vi "GUI Set Error and Display Error Status.vi"(1 "error in":errorcluster, 2 "Write status only if error occures? (False)":bool, 3 "error name (error)":string="error", 4 "status string name (stat1)":string="stat1") -> ()   [LabVIEW 2013]
doc: "GUI helper: Takes value of error line, sets it to named error indicator and writes either 'READY' or 'ERROR' to the named status string. Both error and status string indicator must be registered by SGUI lib before this can be used."
uses:
  varilib/SGUI Assign Multiple Strings With Tags By Label.vi
  varilib/varilib.lvlib
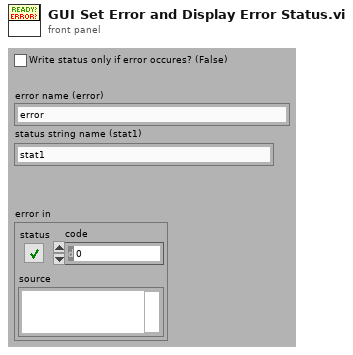
[diagram p1: front panel]
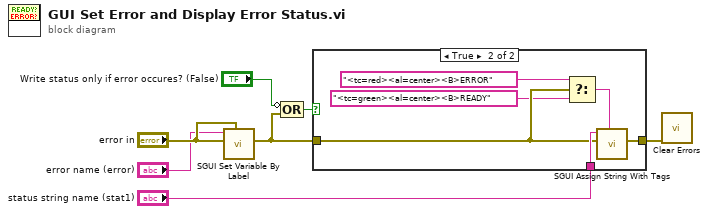
[diagram p0: block diagram]
diagram:
  n1 = call "SGUI Set Variable By Label.vi"("value (none)"="error in", "error in"="error in", "control label (none)"="error name (error)") -> ("error out"=w3:errorcluster)  [unwired: 7 in, 1 out]
  n2 = Compound Arithmetic op=OR(invert "Write status only if error occures? (False)", w3) -> (w1:bool)
  n3 = case shown="True" w1 {
    tunnel: "status string name (stat1)" -> [_ w14]
    tunnel: w3 -> [w8 w13]
    tunnel: [w8 w11] -> w4
    frame False {
    }
    frame True {
      n4 = Select(t="<tc=red><al=center><B>ERROR", s=w13, f="<tc=green><al=center><B>READY") -> (s? t:f=w12:string)
      n5 = call-poly "SGUI Assign String With Tags.vi"("error in"=w13, "label(s) (empty)"=w14, "string (empty)"=w12) -> ("error out"=w11:errorcluster)  [unwired: 7 in, 1 out]
    }
  }
  n6 = call <vilib>:"Clear Errors.vi"("error in (no error)"=w4) -> ()  [unwired: 6 in, 1 out]
